vi "inspector_scale_y.vi"(7 "error in":errorcluster, 8 "Borders":T1, 9 "Waveform in":cluster{dbl, dbl, "Data out":dbl[]}, 10 "Overview Graph in":refnum<vi>) -> (0 "error out":errorcluster, 3 "Overview Graph out":refnum<vi>)   [LabVIEW 2010]
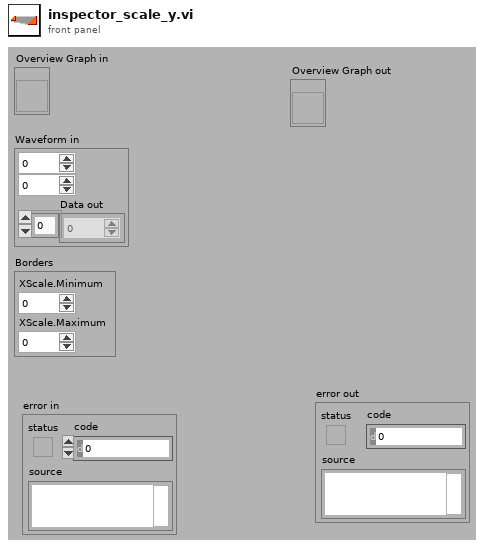
[diagram p1: front panel]
types:
  T1 = cluster{"XScale.Minimum":dbl, "XScale.Maximum":dbl}
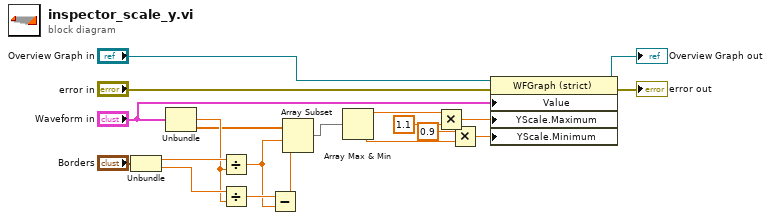
[diagram p0: block diagram]
diagram:
  n1 = Unbundle("Borders") -> ("XScale.Minimum"=w8:dbl, "XScale.Maximum"=w7:dbl)
  n2 = Unbundle("Waveform in") -> (w6:dbl, "Data out"=w5:dbl[])  [unwired: 1 out]
  n3 = Divide(x=w8, y=w6) -> (x/y=w3:dbl)
  n4 = Divide(x=w7, y=w6) -> (x/y=w4:dbl)
  n5 = Subtract(x=w4, y=w3) -> (x-y=w2:dbl)
  n6 = Array Subset(array=w5, index=w3, length=w2) -> (w1:dbl[])
  n7 = Array Max & Min(array=w1) -> (max value=w11:dbl, min value=w15:dbl)  [unwired: 2 out]
  n8 = Multiply(x=w11, y=1.1) -> (x*y=w12:dbl)
  n9 = Multiply(x=0.9, y=w15) -> (x*y=w13:dbl)
  n10 = property class="WFGraph (strict)"(reference="Overview Graph in", error in="error in", "Value"="Waveform in", "YScale.Maximum"=w12, "YScale.Minimum"=w13) -> (reference out=→"Overview Graph out":refnum<vi>, error out=→"error out":errorcluster)
